vi "filter tags available for mapping to channel.vi"(10 "channel to map to":refnum<class "TBM channel.lvclass">, 11 "engine configuration in":refnum<class "engine configuration.lvclass">) -> (2 "filtered tags":refnum<class "tag descriptor.lvclass">[](array[class]), 3 "engine configuration out":refnum<class "engine configuration.lvclass">)   [LabVIEW 2013, in "engine configuration.lvclass"]
uses:
  engine configuration.lvclass
  <vilib>/NI/Tag Bus Module Framework/channel/TBM channel.lvclass
  <vilib>/NI/Tag Bus/tag/tag descriptor.lvclass
  <vilib>/NI/Tag Bus Module Framework/channel/TBM channel.lvclass/TBM channel.ctl
  engine configuration.lvclass/engine configuration.ctl
  <vilib>/NI/Tag Bus/tag/tag descriptor.lvclass/tag descriptor.ctl
  <vilib>/NI/Tag Bus Module Framework/channel/Read channel classification.vi
  <vilib>/NI/Tag Bus/tag/read data type.vi
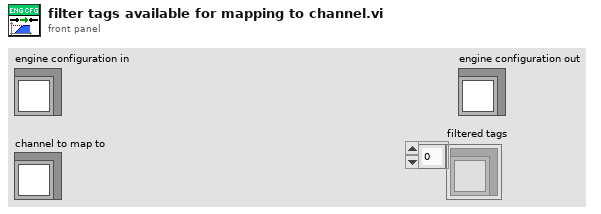
[diagram p1: front panel]
types:
  T1 = typedef "TBM channel.lvclass/channel classification.ctl" = enum16{"input data", "output data", "processing parameter", "processing result"}
  T2 = typedef "tag bus.lvlib/tag descriptor.lvclass/Data Type.ctl" = enum16{"Double", "Single", "I64", "I32", "I16", "I8", "U64", "U32", "U16", "U8", "Boolean", "String", "Array of Double", "Array of Single", "Array of I64", "Array of I32", "Array of I16", "Array of I8", "Array of U64", "Array of U32", "Array of U16", "Array of U8", "Array of Boolean", "Array of String"}
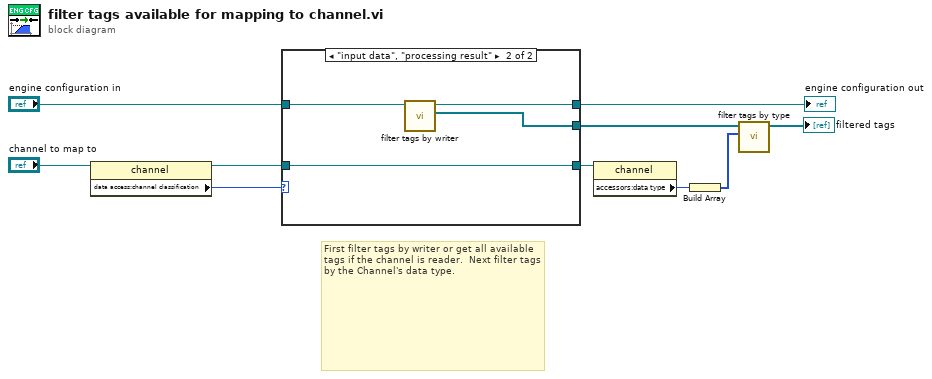
[diagram p0: block diagram]
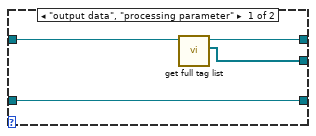
[diagram p2: hidden frame]
diagram:
  # "First filter tags by writer or get all available tags if the channel is reader.  Next filter tags by the Channel's data type."
  n1 = property class="channel"(reference="channel to map to") -> (reference out=w7:refnum<class "TBM channel.lvclass">, "data access:channel classification"=w9:T1)  [unwired: 1 in, 1 out]
  n2 = case shown="\"input data\", \"processing result\"" w9 {
    tunnel: "engine configuration in" -> [w13 w18]
    tunnel: w7 -> [w14 w15]
    tunnel: [w14 w15] -> w5
    tunnel: [w12 w17] -> w6
    tunnel: [w11 w16] -> w4
    frame "output data", "processing parameter" {
      n3 = call "get full tag list.vi"("engine configuration in"=w13) -> ("tag list"=w11:refnum<class "tag descriptor.lvclass">[], "engine configuration out"=w12:refnum<class "engine configuration.lvclass">)  [unwired: 9 in]
    }
    frame "input data", "processing result" {
      n4 = call "filter tags by writer.vi"("engine configuration in"=w18) -> ("tag list"=w16:refnum<class "tag descriptor.lvclass">[], "engine configuration out"=w17:refnum<class "engine configuration.lvclass">)  [unwired: 9 in]
    }
  }
  "engine configuration out" <- w6
  n5 = property class="channel"(reference=w5) -> ("accessors:data type"=w3:T2)  [unwired: 1 in, 2 out]
  n6 = Build Array(w3) -> (w2:T2[])
  n7 = call <vilib>:"filter tags by type.vi"("allowable types"=w2, "tags in"=w4) -> ("filtered tags"=→"filtered tags":refnum<class "tag descriptor.lvclass">[])  [unwired: 9 in]
